vi "Excimer shot on demand-timed V3.vi"() -> ()   [LabVIEW 2019]
doc: "This example demonstrates how to generate a finite amount of data from a buffer in your computer's memory."
uses:
  <resource>/objmgr/daqmx.rc
  <vilib>/DAQmx/configure/timing.llb/DAQmx Timing (Sample Clock).vi
  <vilib>/DAQmx/create/channels.llb/DAQmx Create Channel (AO-Voltage-Basic).vi
  <vilib>/Utility/error.llb/DialogType.ctl
  <vilib>/DAQmx/write.llb/DAQmx Write (Analog 1D Wfm NChan NSamp).vi
  <vilib>/DAQmx/configure/trigger.llb/DAQmx Start Trigger (Digital Edge).vi
panel:
  out "error out - Stop":errorcluster
  in  "Digital Start Trigger Edge":i32(ring)=10280 caption="Edge" items=["Rising"=10280, "Falling"=10171]
  in  "Digital Start Trigger Source":tag="/Dev1/PFI0" caption="Source"
  in  "trig time/ms":dbl=1.0
  out "Waveform\nsize":i32
  out "SampPerChan":dbl
  in  "magnetron cycle/ms":dbl=2.0
  out "error out - Setup":errorcluster
  out "Loop counter":i32=14
  in  "stop":bool
  in  "Number of Shots":dbl=2.0
  out "Waveform Graph":waveform(dbl)[](graph)=[{"t0"=timestamp(0 s since 1904-01-01), "dt"=0.001, "Y"=[5.0, 5.0, 5.0, 5.0, 5.0, 5.0, 5.0, 5.0, 5.0, 5.0, 5.0, 5.0, 5.0, 5.0, 5.0, 5.0, 5.0, 5.0, 5.0, 5.0, 5.0, 5.0, 5.0, 5.0, 5.0, 5.0, 5.0, 5.0, 5.0, 5.0, 5.0, 5.0, 5.0, 5.0, 5.0, 5.0, 5.0, 5.0, 5.0, 5.0, 5.0, 5.0, 5.0, 5.0, 5.0, 5.0, 5.0, 5.0, 5.0, 5.0, 0.0, 0.0, 0.0, 0.0, 0.0, 0.0, 0.0, 0.0, 0.0, 0.0, 0.0, 0.0, 0.0, 0.0, 0.0, 0.0, 0.0, 0.0, 0.0, 0.0, 0.0, 0.0, 0.0, 0.0, 0.0, 0.0, 0.0, 0.0, 0.0, 0.0, 0.0, 0.0, 0.0, 0.0, 0.0, 0.0, 0.0, 0.0, 0.0, 0.0, 0.0, 0.0, 0.0, 0.0, 0.0, 0.0, 0.0, 0.0, 0.0, 0.0, 0.0, 0.0, 0.0, 0.0, 0.0, 0.0, 0.0, 0.0, 0.0, 0.0, 0.0, 0.0, 0.0, 0.0, 0.0, 0.0, 0.0, 0.0, 0.0, 0.0, 0.0, 0.0, 0.0, 0.0, 0.0, 0.0, 0.0, 0.0, 0.0, 0.0, 0.0, 0.0, 0.0, 0.0, 0.0, 0.0, 0.0, 0.0, 0.0, 0.0, 0.0, 0.0, 0.0, 0.0, 0.0, 0.0, 0.0, 0.0, 0.0, 0.0, 0.0, 0.0, 0.0, 0.0, 0.0, 0.0, 0.0, 0.0, 0.0, 0.0, 0.0, 0.0, 0.0, 0.0, 0.0, 0.0, 0.0, 0.0, 0.0, 0.0, 0.0, 0.0, 0.0, 0.0, 0.0, 5.0, 5.0, 5.0, 5.0, 5.0, 5.0, 5.0, 5.0, 5.0, 5.0, 5.0, 5.0, 5.0, 5.0, 5.0, 5.0, 5.0, 5.0, 5.0, 5.0, 5.0, 5.0, 5.0, 5.0, 5.0, 5.0, 5.0, 5.0, 5.0, 5.0, 5.0, 5.0, 5.0, 5.0, 5.0, 5.0, 5.0, 5.0, 5.0, 5.0, 5.0, 5.0, 5.0, 5.0, 5.0, 5.0, 5.0, 5.0, 5.0, 5.0, 0.0, 0.0, 0.0, 0.0, 0.0, 0.0, 0.0, 0.0, 0.0, 0.0, 0.0, 0.0, 0.0, 0.0, 0.0, 0.0, 0.0, 0.0, 0.0, 0.0, 0.0, 0.0, 0.0, 0.0, 0.0, 0.0, 0.0, 0.0, 0.0, 0.0, 0.0, 0.0, 0.0, 0.0, 0.0, 0.0, 0.0, 0.0, 0.0, 0.0, 0.0, 0.0, 0.0, 0.0, 0.0, 0.0, 0.0, 0.0, 0.0, 0.0, 0.0, 0.0, 0.0, 0.0, 0.0, 0.0, 0.0, 0.0, 0.0, 0.0, 0.0, 0.0, 0.0, 0.0, 0.0, 0.0, 0.0, 0.0, 0.0, 0.0, 0.0, 0.0, 0.0, 0.0, 0.0, 0.0, 0.0, 0.0, 0.0, 0.0, 0.0, 0.0, 0.0, 0.0, 0.0, 0.0, 0.0, 0.0, 0.0, 0.0, 0.0, 0.0, 0.0, 0.0, 0.0, 0.0, 0.0, 0.0, 0.0, 0.0, 0.0, 0.0, 0.0, 0.0, 0.0, 0.0, 0.0, 0.0, 0.0, 0.0, 0.0, 0.0, 0.0, 0.0, 0.0, 0.0, 0.0, 0.0, 0.0, 0.0, 0.0, 0.0, 0.0, 0.0, 0.0]}]
  in  "Sample Rate":dbl=1000.0
  in  "Sample Clock Source":tag="OnboardClock"
  in  "Physical Channel(s)":tag="Dev1/ao1"
  out "Actual Sample Rate":dbl=1000.0 format="%0.2f"
  # "Channel Settings"
  # "Output"
  # "Timing and Buffer Settings"
  # "Waveform Settings"
  # "Trigger Settings"
  # "Example for 10Hz Nd:YAG:\nleave sample rate at 1000 for ms timing\nfrequency = 10         \nTrig source = PFI0    physical chanel select as wired e.g. ao1\nedge rising                then set # shots and run\nworks off solariX trigger\nmake sure solariX trig time is total pulse time +0.02"
  # "made to work in ms\nso mag motion and trig time are in integers to correspond with dt of timing"
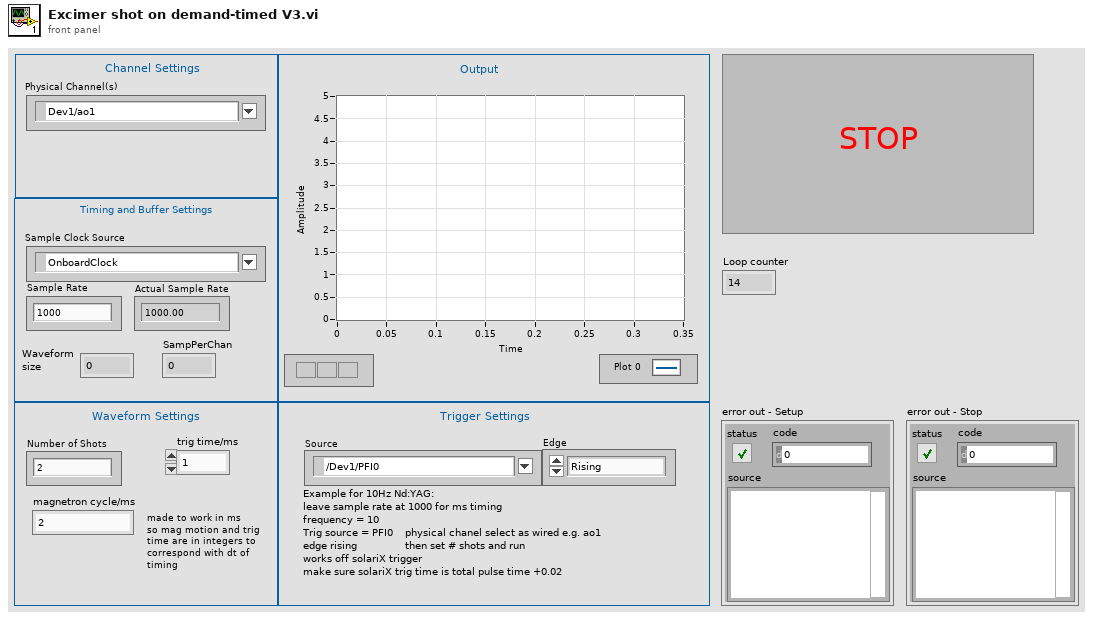
[diagram p1: front panel]
types:
  T1 = typedef "DialogType.ctl" = u16
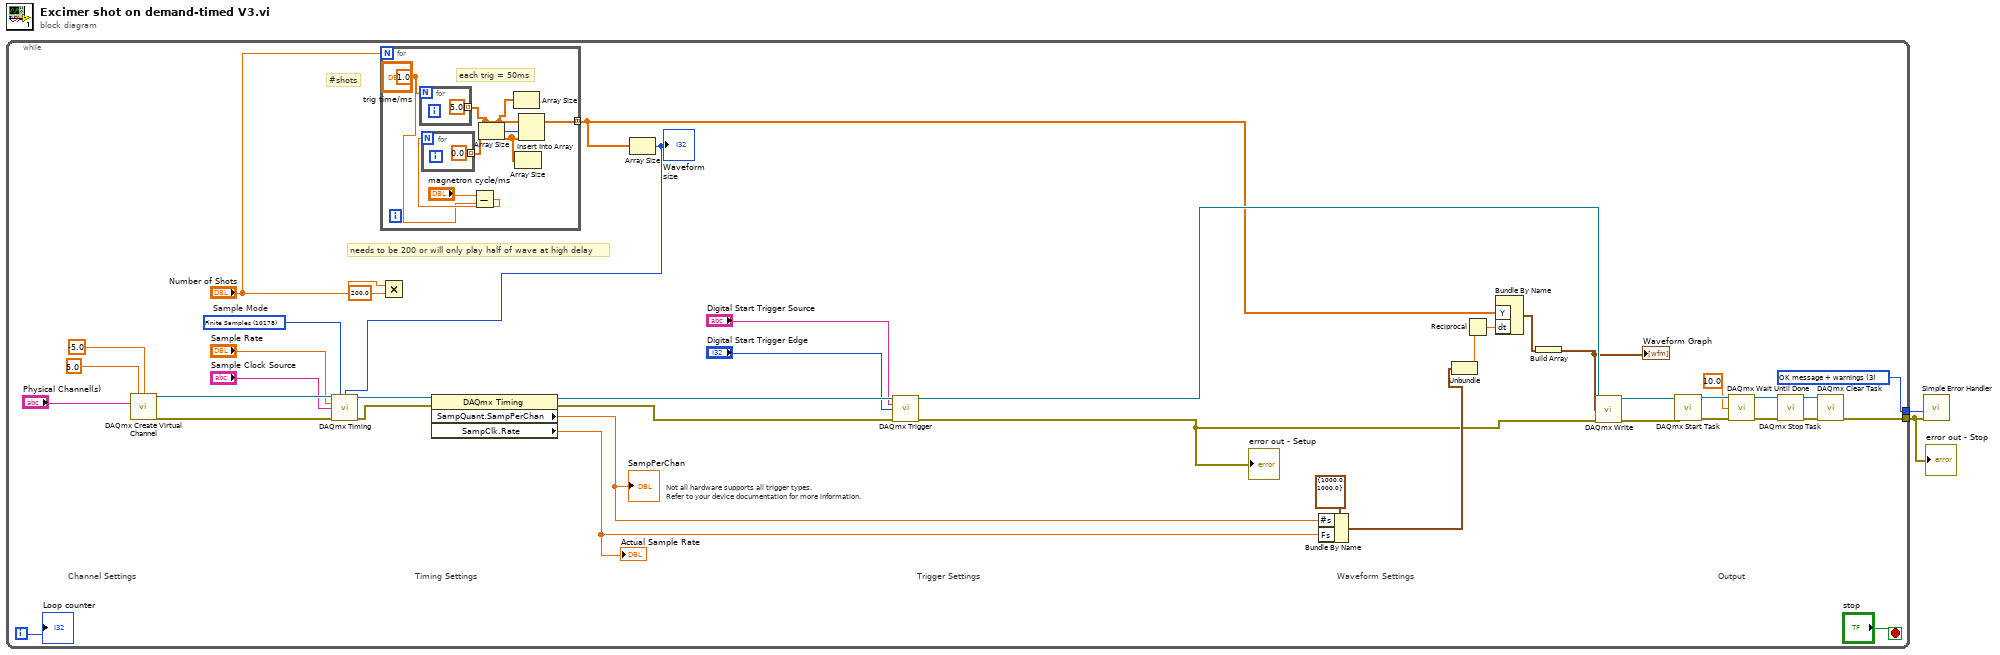
[diagram p0: block diagram]
diagram:
  n1 = while {
    tunnel: [w39] -> w1
    tunnel: [w21] -> w2
    i -> [w15]
    stop <- "stop" stop-if-true
    w21 = T1 3 items=["no dialog", "OK message", "continue or stop message", "OK message + warnings", "continue/stop + warnings"] ("type of dialog (OK msg:1)")
    w42 = 10178 items=["Finite Samples"=10178, "Continuous Samples"=10123, "Hardware Timed Single Point"=12522]  # Sample Mode
    # "needs to be 200 or will only play half of wave at high delay"
    # "#shots"
    # "Trigger Settings"
    # "Not all hardware supports all trigger types.\nRefer to your device documentation for more information."
    # "Output"
    # "Waveform Settings"
    # "Timing Settings"
    # "Channel Settings"
    n2 = call-poly <vilib>:"DAQmx Create Virtual Channel.vi"("maximum value"=5.0 ("Max Voltage"), "minimum value"=-5.0 ("Min Voltage"), "physical channels"="Physical Channel(s)") -> ("task out"=w40:refnum<k21>, "error out"=w41:errorcluster)  [unwired: 11 in]
    n3 = for {
      N: "Number of Shots" -> [_]
      tunnel: [w46] -> w7 mode=concatenating
      w48 = 1.0 ("y")
      # "each trig = 50ms"
      n4 = for {
        N: w48 -> [_]
        tunnel: [5.0] -> w44 mode=indexing
      }
      n5 = Subtract(x="magnetron cycle/ms", y=w48) -> (x-y=w49:dbl)
      n6 = for {
        N: w49 -> [_]
        tunnel: [0.0] -> w45 mode=indexing
      }
      n7 = Array Size(array=w44) -> (size(s)=w47:i32)
      n8 = Array Size(array=w44) -> ()  [unwired: 1 out]
      n9 = Array Size(array=w45) -> ()  [unwired: 1 out]
      n10 = Insert Into Array(array=w44, index=w47, new element=w45) -> (w46:dbl[])
    }
    n11 = Multiply(x="Number of Shots", y=200.0) -> ()  [unwired: 1 out]
    n12 = Array Size(array=w7) -> (size(s)=w6:i32)
    "Waveform\nsize" <- w6
    n13 = call-poly <vilib>:"DAQmx Timing.vi"("task/channels in"=w40, "sample mode"=w42, "samples per channel"=w6, "rate"="Sample Rate", "source"="Sample Clock Source", "error in"=w41) -> ("task out"=w43:refnum<k21>, "error out"=w3:errorcluster)  [unwired: 8 in]
    n14 = property class="DAQmx Timing"(reference=w43, error in=w3) -> (reference out=w18:refnum<k21>, error out=w19:errorcluster, "SampQuant.SampPerChan"=w27:dbl, "SampClk.Rate"=w26:dbl)
    "Actual Sample Rate" <- w26
    "SampPerChan" <- w27
    n15 = call-poly <vilib>:"DAQmx Trigger.vi"("task/channels in"=w18, "source"="Digital Start Trigger Source", "edge"="Digital Start Trigger Edge", "error in"=w19) -> ("task out"=w20:refnum<k21>, "error out"=w11:errorcluster)  [unwired: 10 in]
    "error out - Setup" <- w11
    n16 = Bundle By Name(cluster=cluster{"Fs":dbl, "#s":dbl} {"Fs"=1000.0, "#s"=1000.0} ("sampling info"), "#s"=w27, "Fs"=w26) -> (w32:cluster{"Fs":dbl, "#s":dbl})
    n17 = Unbundle(w32) -> ("Fs"=w9:dbl)  [unwired: 1 out]
    n18 = Reciprocal(x=w9) -> (1/x=w8:dbl)
    n19 = Bundle By Name("Y"=w7, "dt"=w8) -> (w10:waveform(dbl))  [unwired: 1 in]
    n20 = Build Array(w10) -> (w14:waveform(dbl)[])
    "Waveform Graph" <- w14
    n21 = call-poly <vilib>:"DAQmx Write.vi"("task/channels in"=w20, "data"=w14, "error in"=w11) -> ("task out"=w31:refnum<k21>, "error out"=w30:errorcluster)  [unwired: 10 in, 1 out]
    n22 = call <vilib>:"DAQmx Start Task.vi"("task/channels in"=w31, "error in"=w30) -> ("task out"=w29:refnum<k21>, "error out"=w28:errorcluster)  [unwired: 12 in]
    n23 = call <vilib>:"DAQmx Wait Until Done.vi"("task/channels in"=w29, "timeout (sec)"=10.0, "error in"=w28) -> ("task out"=w23:refnum<k21>, "error out"=w22:errorcluster)  [unwired: 11 in]
    n24 = call <vilib>:"DAQmx Stop Task.vi"("task/channels in"=w23, "error in"=w22) -> ("task out"=w25:refnum<k21>, "error out"=w24:errorcluster)  [unwired: 12 in]
    n25 = call <vilib>:"DAQmx Clear Task.vi"("task in"=w25, "error in"=w24) -> ("error out"=w39:errorcluster)  [unwired: 13 in]
    "Loop counter" <- w15
  }
  "error out - Stop" <- w1
  n26 = call <vilib>:"Simple Error Handler.vi"("type of dialog (OK msg:1)"=w2, "error in (no error)"=w1) -> ()  [unwired: 3 in, 5 out]
